vi "Dryer PreCondition SM.vi"(0 "Equipment":T1, 1 "CDAQ Tasks":refnum<k21>[](array[refnum]), 5 "RDB Channel":string="1001", 7 "Power On Threshold":dbl=50.0, 9 "CDAQ?":bool, 11 "Error In":errorcluster) -> (4 "Cold Dryer Weight":dbl, 15 "Error Out":errorcluster)   [LabVIEW 2012]
uses:
  Equipment DPT.ctl
  WT500/WT500 Sequences.ctl
  Global Test Variables DPT.vi
  <vilib>/Analysis/baseanly.llb/Mean (DBL).vi
  Drivers/Agilent 34970/Agilent 34970.lvlib
  <vilib>/Analysis/NI_AALBase.lvlib
panel:
  out "Debug State":string[](array[string])
  in  "Tab Control":enum32{"Page 1", "Page 2"}(tab)
  out "CDAQ Data Out":dbl[](array[numeric])
  out "15 min Up":bool
  out "Temp stable":bool
  out "Current State":string
  in  "Debug?":bool=TRUE
  in  "10 Min":i32=600
  in  "5min":dbl=300.0
  out "Test Setup.RH-IP":string
  out "Test AG Chan List":string
  out "Saved Channel List":string
  out "Agilent Error Message":string
  out "Timer":dbl format="%<%H:%M:%S>t"
  out "Temperature-RDB":dbl(graph)
  out "RDB (F)":dbl
  out "Ambient Temp(F)":dbl
  out "RH":dbl
  out "Power":dbl
  out "String":string
  in  "Exit":bool
  # "Before any test cycle, operate the dryer without a test load in the non-heat mode for 15 minutes\nor until the discharge air temperature is varying less than 1 °F for 10 minutes, which ever is longer, in the test installation location\nwith the ambient conditions within the specified rest condition tolerances of 2.2."
  # "2.2 Ambient temperature and humidity. Maintain the room ambient air temperature at 75 ±3 °F and the room relative humidity at 50\n±10 percent relative humidity"
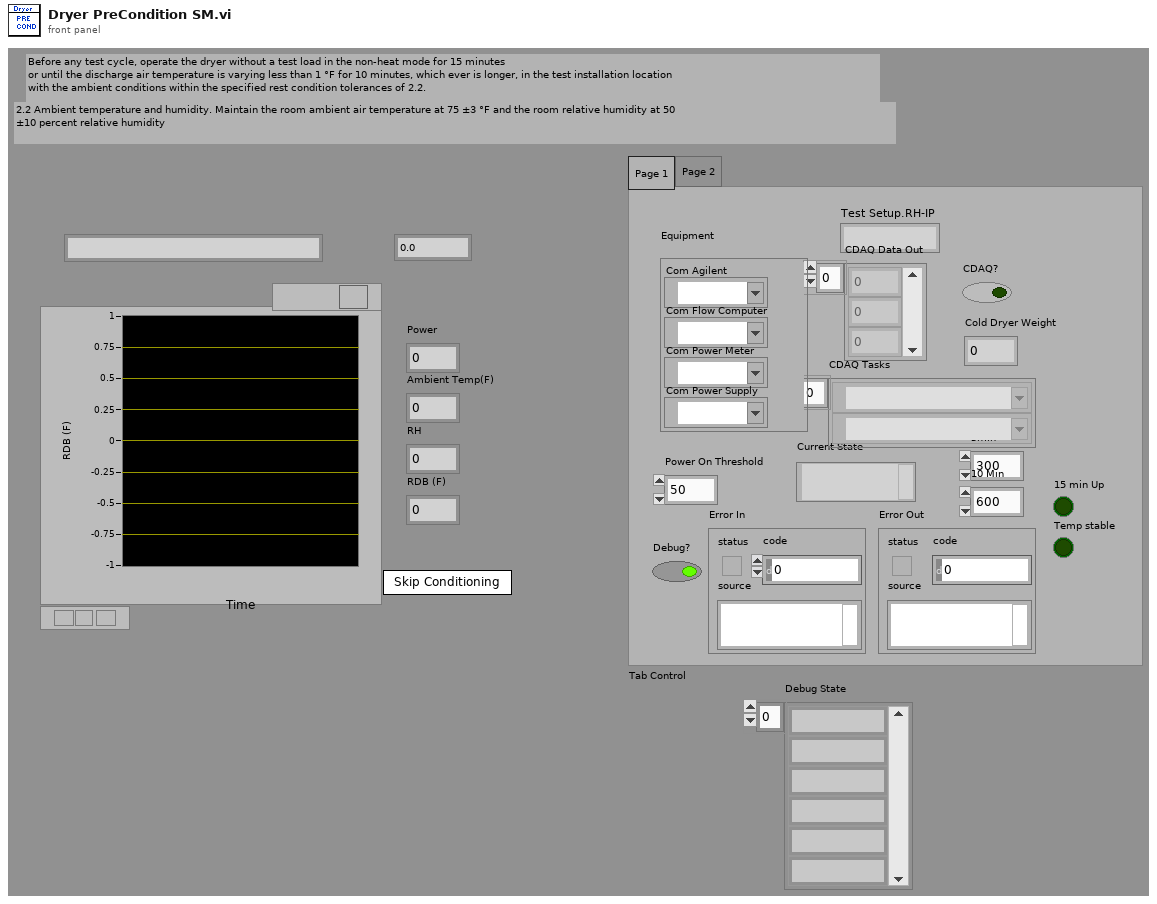
[diagram p1: front panel]
types:
  T1 = typedef "Equipment DPT.ctl" = cluster{"Com Agilent":refnum<visa-resource-name>, "Com Flow Computer":refnum<visa-resource-name>, "Com Power Meter":refnum<visa-resource-name>, "Com Power Supply":refnum<visa-resource-name>}
  T2 = enum32{"invalid app kind", "Development System", "Run Time System", "Student Edition", "Embedded LabVIEW", "Evaluation", "Custom"}
  T3 = enum16{"Exe", "Init CDAQ", "Gather DATA", "Close"}
  T4 = enum32{"Invalid", "Standard", "Closed", "Hidden", "Minimized", "Maximized"}
  T5 = typedef "WT500 Sequences.ctl" = enum16{"Initialize", "GetReadings", "GetErrors", "Close", "NoOp", "MiscCmd"}
  T6 = cluster{"Core":cluster{"Current VI Reference":refnum<vi>, "Close Panel on Exit?":bool}, "Agilent Channel List":string, "Equipment":T1, "Power On Threshold":dbl, "RDB Channel":string, "T0":dbl, "Tstart":dbl, "Temps":dbl[], "CDAQ?":bool, "CDAQ Tasks":refnum<k21>[]}
  T7 = cluster{"Current VI Reference":refnum<vi>, "Close Panel on Exit?":bool}
  T8 = typedef "DPT Global Type.ctl" = cluster{"Test Setup":cluster{"RH Resistor":dbl, "Temp Cal":dbl, "Temp Coeff":dbl, "Power On Threshold":dbl, "MA Filter Size":i32, "Weight Offset":dbl, "Temp Resistor":dbl, "Gas Enabled":bool, "Gas P. Resistor":dbl, "Scale Com":dbl, "W. Samps":i32, "Temp4mA Val":dbl, "Temp20mA Val":dbl, "RH4mA Val":dbl, "RH20mA Val":dbl, "GPres4mA Val":dbl, "Gpres20mA Val":dbl, "Smoothing":bool, "CDAQ":bool, "34970":bool, "34980":bool, "RH-IP":string, "RH-IP2":string, "RH-IP3":string, "CompVolume":dbl, "T45_Coeff.":dbl}, "Agilent Setup":cluster{"Scale Channel":string, "TC Channels":string, "VDC Discrete Channels":string, "RH Chan":string, "Temp Chan":string, "Tscale Channel":string, "RDB Channel":string, "Gas Temperature":string, "Gas Pressure":string, "Barometric Pressure":string, "Gas Feedback Chan":string}, "Directories":cluster{"Work File Directory":path, "Save File Directory":path, "Library Directory":path, "Data Backup Directory":path, "Data Backup Dir Fail":path, "Lab Directory":path}, "Test Information":cluster{"Model:":string, "Temperature:":string, "Engineer:":string, "Technician:":string, "Comments:":string, "Lab ID:":string, "TR Number:":string, "Test Number:":string, "Test Station:":string, "Empty Dryer Cold Weight:":dbl, "Serial Number:":string, "Build:":string, "Dryer Type":string, "Humidity":string, "Test Title per TR:":string}, "cDAQ Array Locations":cluster{"Scale Channel":string, "TC Channels":string, "VDC Discrete Channel":string, "RH Chan":string, "Temp Chan":string, "Tscale Channel":string, "RDB Channel":string, "Gas Temperature":string, "Gas Pressure":string, "Barometric Pressure":string, "Gas Feedback Chan":string}}
  T9 = typedef "Dryer PowerData.ctl" = cluster{"Current L1":dbl, "Current L2":dbl, "Power":dbl, "WattHours":dbl}
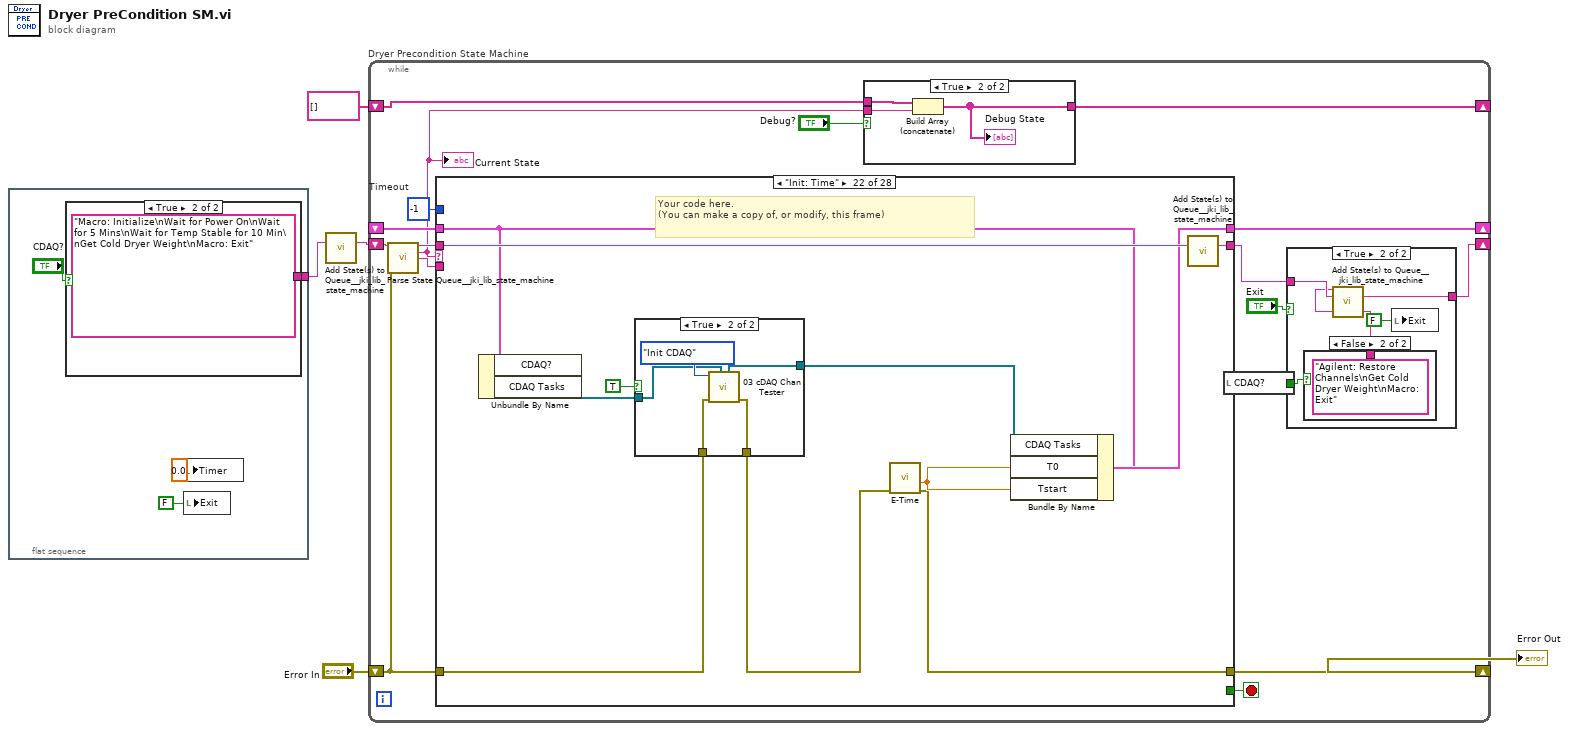
[diagram p0: block diagram]
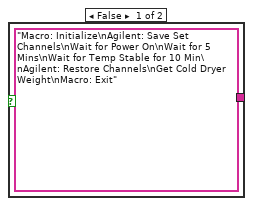
[diagram p2: hidden frame]
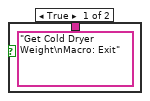
[diagram p5: hidden frame]
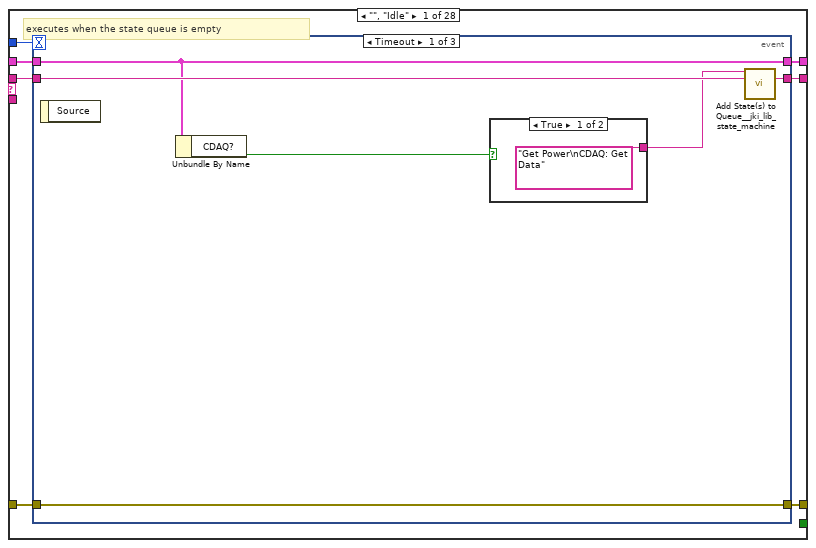
[diagram p6: hidden frame]
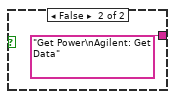
[diagram p7: hidden frame]
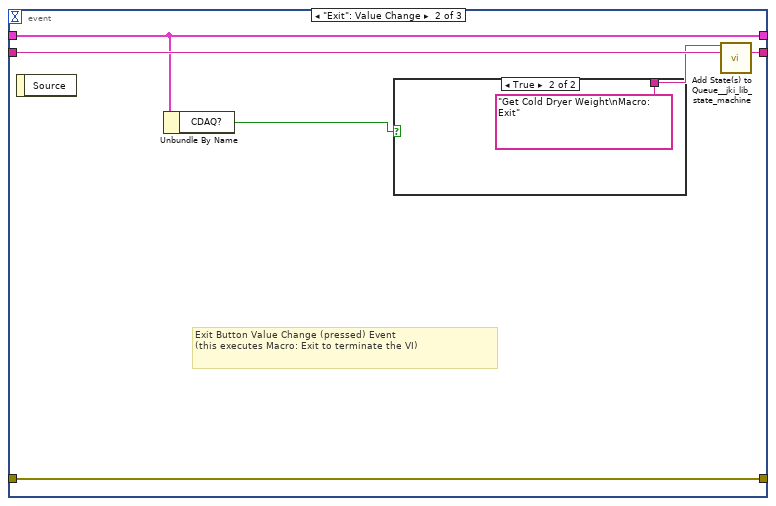
[diagram p8: hidden frame]
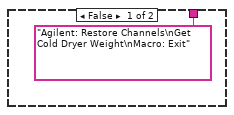
[diagram p9: hidden frame]
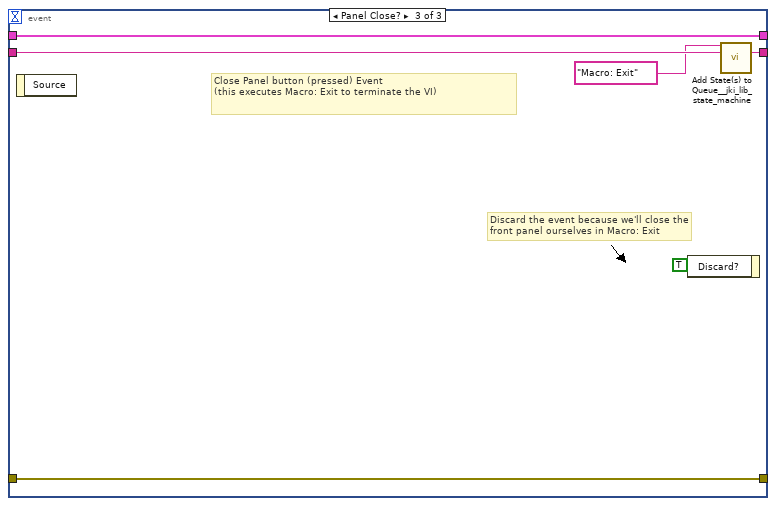
[diagram p10: hidden frame]
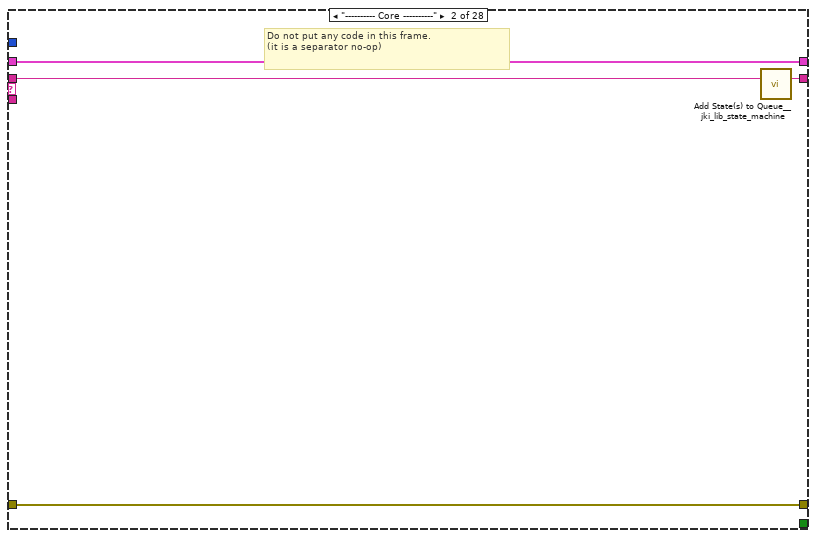
[diagram p11: hidden frame]
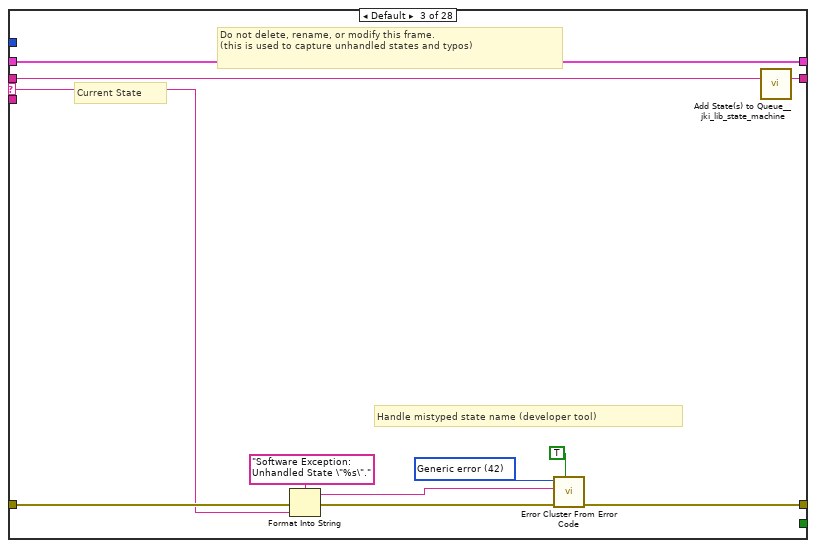
[diagram p12: hidden frame]
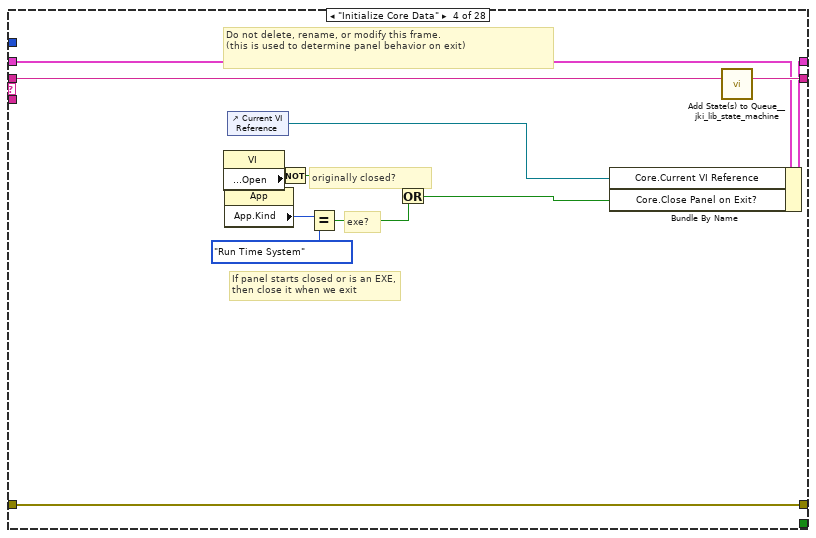
[diagram p13: hidden frame]
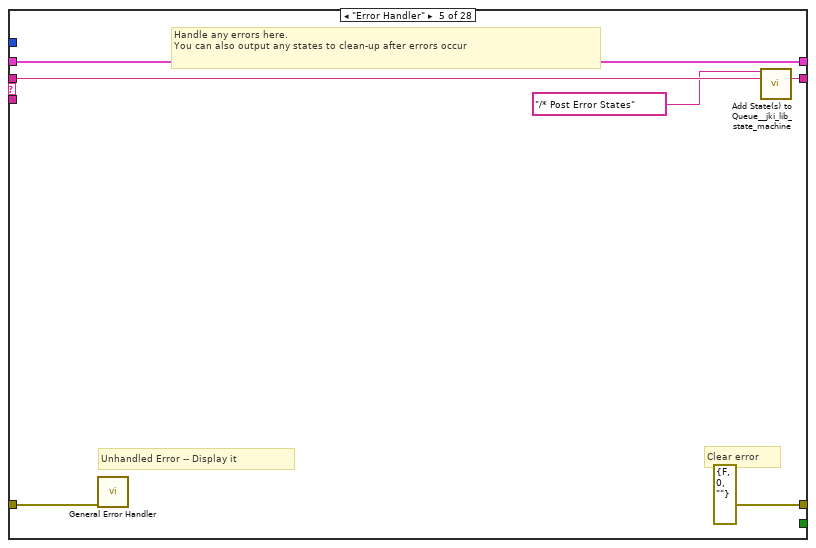
[diagram p14: hidden frame]
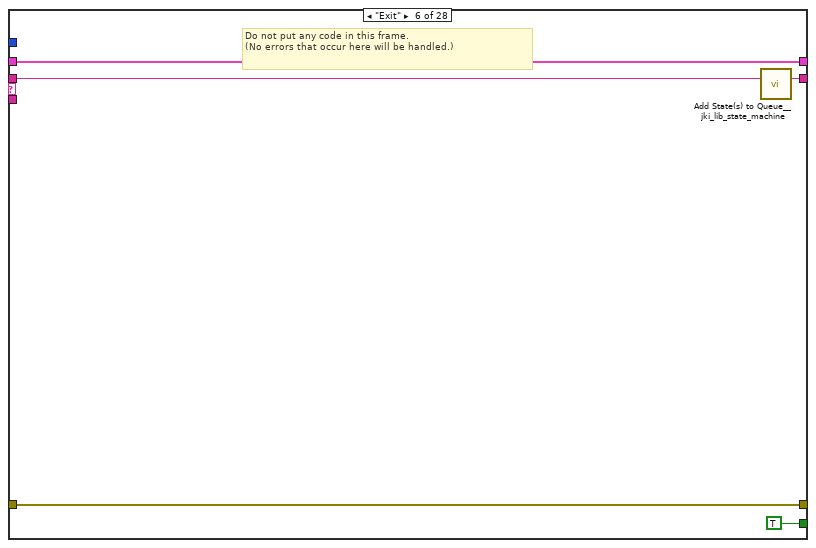
[diagram p15: hidden frame]
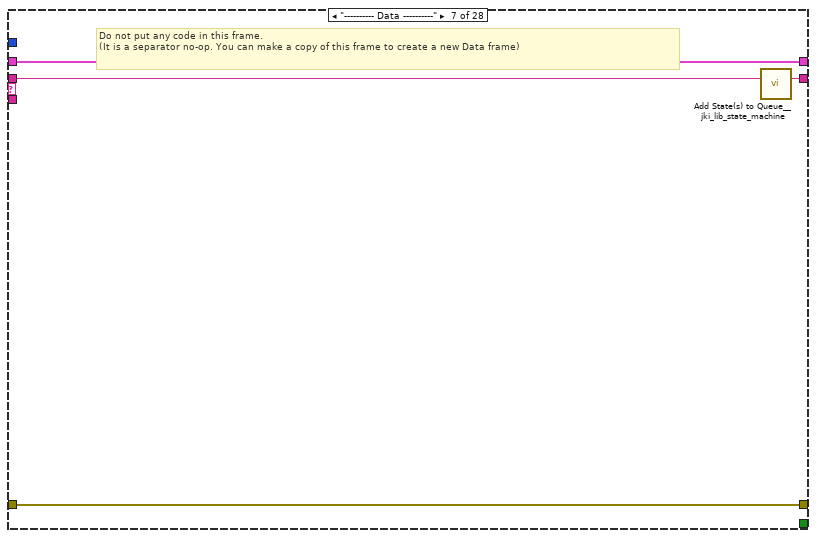
[diagram p16: hidden frame]
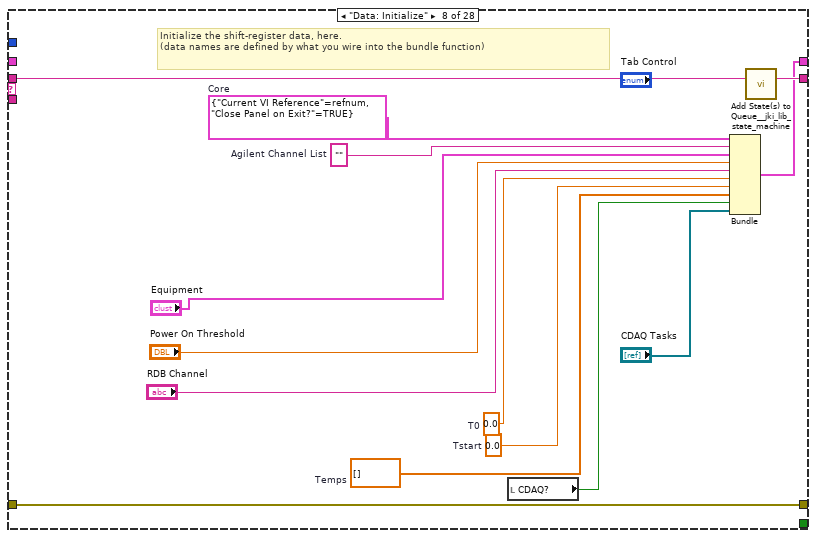
[diagram p17: hidden frame]
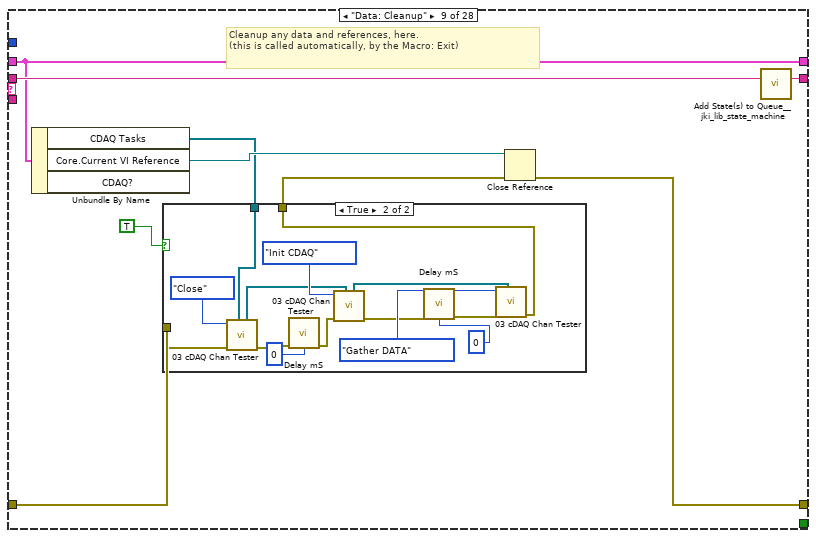
[diagram p18: hidden frame]
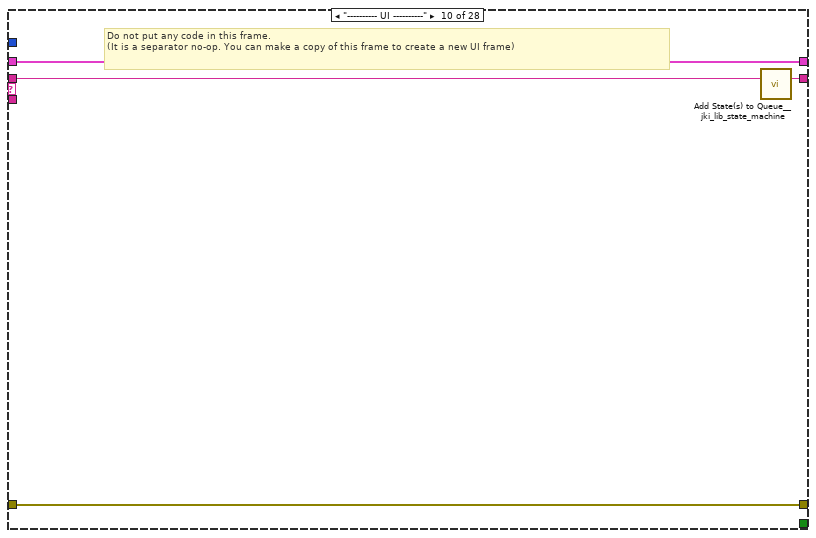
[diagram p20: hidden frame]
diagram:
  n1 = flat-sequence {
    tunnel: [w9] -> w4
    frame #0 {
      n2 = case shown="True" "CDAQ?" {
        tunnel: ["Macro: Initialize\nAgilent: Save Set Channels\nWait for Power On\nWait for 5 Mins\nWait for Temp Stable for 10 Min\nAgilent: Restore Channels\nGet Cold Dryer Weight\nMacro: Exit" "Macro: Initialize\nWait for Power On\nWait for 5 Mins\nWait for Temp Stable for 10 Min\nGet Cold Dryer Weight\nMacro: Exit"] -> w9
        frame False {
        }
        frame True {
        }
      }
      n3 = local write "Timer"(0.0 ("Timer")) -> ()
      n4 = local write "Exit"(FALSE ("Exit")) -> ()
    }
  }
  n5 = call <vilib>:"Add State(s) to Queue__jki_lib_state_machine.vi"("State(s) in (\"\")"=w4) -> ("States Out"=w5:string)  [unwired: 14 in]
  n6 = while "Dryer Precondition State Machine" {
    shift-right: [w23] -> _
    shift-left: _ -> [w22]
    shift-right: [w25] -> w2
    shift-left: "Error In" -> [w20]
    shift-right: [w18] -> _
    shift-left: w5 -> [w26]
    shift-right: [w13] -> _
    shift-left: string[] [] -> [w12]
    stop <- w24 stop-if-true
    w21 = -1  # Timeout
    n7 = call <vilib>:"Parse State Queue__jki_lib_state_machine.vi"("State Queue"=w26, "Error In (no error)"=w20) -> ("Remaining States"=w28:string, "Current State"=w14:string, "Arguments"=w27:string)  [unwired: 11 in]
    "Current State" <- w14
    n8 = case shown="\"Init: Time\"" w14 {
      selector: w14 -> [_ _ w74 _ _ _ _ _ _ _ _ _ _ _ _ _ _ _ _ _ _ _ _ _ _ _ _ _]
      tunnel: w28 -> [w47 w73 w78 w96 w102 w107 w111 w125 w134 w153 w157 w163 w174 w200 w205 w215 w219 w231 w260 w290 w343 w371 w387 w410 w481 w497 w509 w516]
      tunnel: w27 -> [_ _ _ _ _ _ _ _ _ _ _ w158 w168 _ _ _ _ _ _ _ _ _ _ _ _ _ _ _]
      tunnel: w22 -> [w45 w70 w76 w87 w99 w105 w108 _ w130 w150 w155 w161 w170 w197 w202 w212 w216 w227 w257 w287 w334 w366 w383 w406 w466 w495 w502 w514]
      tunnel: [w44 w71 w80 w93 errorcluster {"status"=FALSE, "code"=0, "source"=""} ("error out") w104 w109 w123 w131 w151 w154 w159 w171 w198 w203 w213 w217 w228 w258 w288 w330 w367 w384 w397 w464 w493 w503 w510] -> w25
      tunnel: w20 -> [w43 w71 w79 w93 w98 w104 w109 w123 w129 w151 w154 w160 w172 w198 w203 w213 w217 w228 w258 w288 w333 w365 w385 w405 w479 w494 w504 w510]
      tunnel: [w46 w72 w77 w95 w101 w106 w110 w124 w133 w152 w156 w162 w173 w199 w204 w214 w218 w230 w259 w289 w342 w370 w386 w409 w480 w496 w508 w515] -> w19
      tunnel: [_ _ _ _ _ TRUE _ _ _ _ _ _ _ _ _ _ _ _ _ _ _ _ _ _ _ _ _ _] -> w24
      tunnel: [w42 w70 w76 w94 w99 w105 w108 w118 w130 w150 w155 w161 w170 w197 w202 w212 w216 w226 w256 w286 w336 w369 w383 w406 w466 w495 w502 w514] -> w23
      tunnel: w21 -> [w41 _ _ _ _ _ _ _ _ _ _ _ _ _ _ _ _ _ _ _ _ _ _ _ _ _ _ _]
      frame "", "Idle" {
        # "executes when the state queue is empty"
        n9 = event shown="[0] Timeout" {
          selector: _ -> [_ _ _]
          dyn-events: _ -> [_ _ _]
          timeout: w41 -> [_ _ _]
          tunnel: w47 -> [w53 w61 w69]
          tunnel: [w52 w60 w68] -> w46
          tunnel: w45 -> [w49 w57 w66]
          tunnel: [w51 w59 w67] -> w44
          tunnel: w43 -> [w51 w59 w67]
          tunnel: [w49 w57 w66] -> w42
          event Timeout {
            n10 = event-data() -> ()  [unwired: 1 in, 1 out]
            n11 = Unbundle By Name(w49) -> ("CDAQ?"=w48:bool)
            n12 = case shown="True" w48 {
              tunnel: ["Get Power\nCDAQ: Get Data" ("State(s) in Front (\"\")") "Get Power\nAgilent: Get Data" ("State(s) in Front (\"\")")] -> w50
              frame True {
              }
              frame False {
              }
            }
            n13 = call <vilib>:"Add State(s) to Queue__jki_lib_state_machine.vi"("State(s) in Front (\"\")"=w50, "State(s) in (\"\")"=w53) -> ("States Out"=w52:string)  [unwired: 13 in]
          }
          event "Exit": Value Change {
            # "Exit Button Value Change (pressed) Event\n(this executes Macro: Exit to terminate the VI)"
            n14 = event-data() -> ()  [unwired: 1 in, 1 out]
            n15 = Unbundle By Name(w57) -> ("CDAQ?"=w56:bool)
            n16 = case shown="True" w56 {
              tunnel: ["Agilent: Restore Channels\nGet Cold Dryer Weight\nMacro: Exit" "Get Cold Dryer Weight\nMacro: Exit"] -> w58
              frame False {
              }
              frame True {
              }
            }
            n17 = call <vilib>:"Add State(s) to Queue__jki_lib_state_machine.vi"("State(s) in Front (\"\")"=w58, "State(s) in (\"\")"=w61) -> ("States Out"=w60:string)  [unwired: 13 in]
          }
          event Panel Close? {
            # "Discard the event because we'll close the front panel ourselves in Macro: Exit"
            # "Close Panel button (pressed) Event\n(this executes Macro: Exit to terminate the VI)"
            n18 = event-data() -> ()  [unwired: 1 in, 1 out]
            n19 = event-data("Discard?"=TRUE) -> ()  [unwired: 1 in, 1 out]
            n20 = call <vilib>:"Add State(s) to Queue__jki_lib_state_machine.vi"("State(s) in Front (\"\")"="Macro: Exit", "State(s) in (\"\")"=w69) -> ("States Out"=w68:string)  [unwired: 13 in]
          }
        }
      }
      frame "---------- Core ----------" {
        # "Do not put any code in this frame.\n(it is a separator no-op)"
        n21 = call <vilib>:"Add State(s) to Queue__jki_lib_state_machine.vi"("State(s) in (\"\")"=w73) -> ("States Out"=w72:string)  [unwired: 14 in]
      }
      frame Default {
        w83 = 42 items=["No error", "Argument error", "Memory is full", "Out of zone", "End of file", "File already open", "Generic file I/O error", "File not found", "File permission error", "Disk is full", "Duplicate path", "Too many files open", "System feature not enabled", "Resource file not found", "Cannot add resource", "Resource not found", "Image not found", "Image memory error", "Pen does not exist", "Config type invalid", "Config token not found", "Config parse error", "Config memory error", "Bad external code format", "Bad external code offset", "External code not present", "Null window", "Destroy window error", "Null menu", "Print aborted", "Bad print record", "Print driver error", "Windows error during printing", "Memory error during printing", "Print dialog error", "Generic print error", "Invalid device refnum", "Device not found", "Device parameter error", "Device unit error", "Cannot open device", "Device call aborted", "Generic error", "Cancelled by user", "Object ID too low", "Object ID too high", "Object not in heap", "Unknown heap", "Unknown object (invalid DefProc)", "Unknown object (DefProc not in table)", "Message out of range", "Invalid (null) method", "Unknown message", "Manager call not supported", "Bad address", "Network operation in progress", "Network operation timed out", "Connection is busy", "Network attribute not supported", "Network error", "Address in use", "System out of memory", "Connection aborted", "Connection refused", "Not connected", "Already connected", "Connection closed", "Initialization error (interapplication manager)", "Bad occurrence", "Wait on unbound occurrence handler", "Occurrence queue overflow", "Datalog type conflict", "Unused", "Unrecognized type (interapplication manager)", "Memory corrupt", "Failed to make temporary DLL", "Old CIN version", "Drag socket not found", "Failed to load drop-object", "Failed to register OLE object", "Failed to release OLE object", "Format specifier type mismatch", "Unknown format specifier", "Too few format specifiers", "Too many format specifiers", "Scan failed", "Newer CIN version", "Error converting to variant", "Runtime menu error", "Password tampered", "Variant attribute not found", "Incompatible variant data type", "Event data is not available", "Event Store is not present", "Occurrence is not found", "Event Queue is not created", "Event info is not available", "Refnum passed is NULL", "Error retrieving Class GUID", "Error retrieving CoClass GUID", "Error retrieving TypeLib GUID.", "Bad built application magic bytes.", "Specific driver is different from the specific driver associated with the Logical Name.", "There is no session opened to the class driver.", "Max Error", "MAX - Error with config objects", "MAX - Error loading configuration", "MAX - Group not supported"]
        # "Current State"
        # "Do not delete, rename, or modify this frame.\n(this is used to capture unhandled states and typos)"
        # "Handle mistyped state name (developer tool)"
        n22 = Format Into String(format string="Software Exception: Unhandled State \"%s\"." ("message"), error in=w79, w74) -> (resulting string=w82:string, error out=w81:errorcluster)  [unwired: 1 in]
        n23 = call <vilib>:"Error Cluster From Error Code.vi"("show call chain? (False)"=TRUE, "error in (no error)"=w81, "error message (\"\")"=w82, "error code (0)"=w83) -> ("error out"=w80:errorcluster)  [unwired: 5 in]
        n24 = call <vilib>:"Add State(s) to Queue__jki_lib_state_machine.vi"("State(s) in (\"\")"=w78) -> ("States Out"=w77:string)  [unwired: 14 in]
      }
      frame "Initialize Core Data" {
        # "Do not delete, rename, or modify this frame.\n(this is used to determine panel behavior on exit)"
        # "originally closed?"
        # "exe?"
        # "If panel starts closed or is an EXE, then close it when we exit"
        n25 = property class="VI"() -> ("Front Panel.Open"=w92:bool)  [unwired: 2 in, 2 out]
        n26 = property class="App"() -> ("App.Kind"=w91:T2)  [unwired: 2 in, 2 out]
        n27 = control-ref of="Current VI Reference"() -> (w85:refnum<vi>)
        n28 = Not(x=w92) -> (.not. x?=w89:bool)
        n29 = Equal?(x=w91, y=T2."Run Time System" ("Application:Kind")) -> (x = y?=w88:bool)
        n30 = Or(x=w89, y=w88) -> (x .or. y?=w86:bool)
        n31 = Bundle By Name(cluster=w87, "Core.Current VI Reference"=w85, "Core.Close Panel on Exit?"=w86) -> (w94:T6)
        n32 = call <vilib>:"Add State(s) to Queue__jki_lib_state_machine.vi"("State(s) in (\"\")"=w96) -> ("States Out"=w95:string)  [unwired: 14 in]
      }
      frame "Error Handler" {
        # "Unhandled Error -- Display it"
        # "Handle any errors here.\nYou can also output any states to clean-up after errors occur"
        # "Clear error"
        n33 = call <vilib>:"General Error Handler.vi"("error in (no error)"=w98) -> ()  [unwired: 10 in, 5 out]
        n34 = call <vilib>:"Add State(s) to Queue__jki_lib_state_machine.vi"("State(s) in Front (\"\")"="/* Post Error States", "State(s) in (\"\")"=w102) -> ("States Out"=w101:string)  [unwired: 13 in]
      }
      frame "Exit" {
        # "Do not put any code in this frame.\n(No errors that occur here will be handled.)"
        n35 = call <vilib>:"Add State(s) to Queue__jki_lib_state_machine.vi"("State(s) in (\"\")"=w107) -> ("States Out"=w106:string)  [unwired: 14 in]
      }
      frame "---------- Data ----------" {
        # "Do not put any code in this frame.\n(It is a separator no-op. You can make a copy of this frame to create a new Data frame)"
        n36 = call <vilib>:"Add State(s) to Queue__jki_lib_state_machine.vi"("State(s) in (\"\")"=w111) -> ("States Out"=w110:string)  [unwired: 14 in]
      }
      frame "Data: Initialize" {
        w114 = dbl[] []  # Temps
        w115 = 0.0  # Tstart
        w116 = 0.0  # T0
        w119 = ""  # Agilent Channel List
        w122 = T7 {"Current VI Reference"=refnum, "Close Panel on Exit?"=TRUE}  # Core
        # "Initialize the shift-register data, here.\n(data names are defined by what you wire into the bundle function)"
        n37 = local read "CDAQ?"() -> (w113:bool)
        n38 = Bundle("Core"=w122, "Agilent Channel List"=w119, "Equipment"="Equipment", "Power On Threshold"="Power On Threshold", "RDB Channel"="RDB Channel", "T0"=w116, "Tstart"=w115, "Temps"=w114, "CDAQ?"=w113, "CDAQ Tasks"="CDAQ Tasks") -> (w118:T6)  [unwired: 1 in]
        n39 = call <vilib>:"Add State(s) to Queue__jki_lib_state_machine.vi"("State(s) in (\"\")"=w125) -> ("States Out"=w124:string)  [unwired: 14 in]
      }
      frame "Data: Cleanup" {
        # "Cleanup any data and references, here.\n(this is called automatically, by the Macro: Exit)"
        n40 = Unbundle By Name(w130) -> ("CDAQ Tasks"=w127:refnum<k21>[], "Core.Current VI Reference"=w132:refnum<vi>)  [unwired: 1 out]
        n41 = case shown="True" TRUE {
          tunnel: w129 -> [w135 w149]
          tunnel: [w135 w140] -> w128
          tunnel: w127 -> [_ w147]
          frame False {
          }
          frame True {
            n42 = call "03 cDAQ Chan Tester.vi"("Tasks In"=w147, "error in (no error)"=w149, "Mode"=T3."Close") -> ("error out"=w145:errorcluster, "Tasks Out"=w142:refnum<k21>[])  [unwired: 6 in, 1 out]
            n43 = call "Delay mS.vi"("Error In"=w145, "milliseconds to wait"=u32 0) -> ("Error Out"=w146:errorcluster)  [unwired: 13 in]
            n44 = call "03 cDAQ Chan Tester.vi"("Tasks In"=w142, "error in (no error)"=w146, "Mode"=T3."Init CDAQ") -> ("error out"=w138:errorcluster, "Tasks Out"=w141:refnum<k21>[])  [unwired: 6 in, 1 out]
            n45 = call "Delay mS.vi"("Error In"=w138, "milliseconds to wait"=u32 0) -> ("Error Out"=w137:errorcluster)  [unwired: 13 in]
            n46 = call "03 cDAQ Chan Tester.vi"("Tasks In"=w141, "error in (no error)"=w137, "Mode"=T3."Gather DATA") -> ("error out"=w140:errorcluster)  [unwired: 6 in, 2 out]
          }
        }
        n47 = Close Reference(reference=w132, error in (no error)=w128) -> (error out=w131:errorcluster)
        n48 = call <vilib>:"Add State(s) to Queue__jki_lib_state_machine.vi"("State(s) in (\"\")"=w134) -> ("States Out"=w133:string)  [unwired: 14 in]
      }
      frame "---------- UI ----------" {
        # "Do not put any code in this frame.\n(It is a separator no-op. You can make a copy of this frame to create a new UI frame)"
        n49 = call <vilib>:"Add State(s) to Queue__jki_lib_state_machine.vi"("State(s) in (\"\")"=w153) -> ("States Out"=w152:string)  [unwired: 14 in]
      }
      frame "UI: Initialize" {
        # "Initialize the User Interface, here.\n(this is called automatically, by the Macro: Init)"
        n50 = call <vilib>:"Add State(s) to Queue__jki_lib_state_machine.vi"("State(s) in (\"\")"=w157) -> ("States Out"=w156:string)  [unwired: 14 in]
      }
      frame "UI: Cursor Set" {
        # "Argument"
        # "Set and Unset Cursor Busy.\n(Usage: \"UI: Cursor Set >> Busy|Idle\")"
        n51 = case shown="\"Idle\", Default" w158 {
          tunnel: w160 -> [w165 w167]
          tunnel: [w164 w166] -> w159
          frame "Idle", Default {
            n52 = call <vilib>:"Unset Busy.vi"("error in (no error)"=w165) -> ("error out"=w164:errorcluster)  [unwired: 10 in]
          }
          frame "Busy" {
            n53 = call <vilib>:"Set Busy.vi"("error in (no error)"=w167) -> ("error out"=w166:errorcluster)  [unwired: 9 in, 1 out]
          }
        }
        n54 = call <vilib>:"Add State(s) to Queue__jki_lib_state_machine.vi"("State(s) in (\"\")"=w163) -> ("States Out"=w162:string)  [unwired: 14 in]
      }
      frame "UI: Front Panel State" {
        # "Argument"
        # "Set Front Panel Open or Closed\n(Usage: \"UI: Front Panel State >> Open|Close\")"
        n55 = Unbundle By Name(w170) -> ("Core.Current VI Reference"=w169:refnum<vi>)
        n56 = case shown="\"Open\", Default" w168 {
          tunnel: w172 -> [w178 w191]
          tunnel: [w180 w192] -> w171
          tunnel: w169 -> [w179 w189]
          frame "Open", Default {
            n57 = property class="VI"(reference=w179, error in=w178) -> (reference out=w176:refnum<vi>, error out=w177:errorcluster, "Front Panel.Open"=w175:bool)
            n58 = case shown="False" w175 {
              tunnel: [w183 w186] -> w180
              tunnel: w177 -> [w182 w186]
              tunnel: w176 -> [w181 _]
              frame False {
                n59 = invoke class="VI" method="FP.Open"(reference=w181, error in=w182, "Activate"=TRUE, "State"=T4."Standard") -> (error out=w183:errorcluster)  [unwired: 1 in, 4 out]
              }
              frame True {
              }
            }
          }
          frame "Close" {
            n60 = property class="VI"(reference=w189, error in=w191) -> (reference out=w188:refnum<vi>, error out=w190:errorcluster, "Front Panel.Open"=w187:bool)
            n61 = case shown="True" w187 {
              tunnel: [w193 w196] -> w192
              tunnel: w190 -> [w193 w195]
              tunnel: w188 -> [_ w194]
              frame False {
              }
              frame True {
                n62 = invoke class="VI" method="FP.Close"(reference=w194, error in=w195) -> (error out=w196:errorcluster)  [unwired: 1 in, 2 out]
              }
            }
          }
        }
        n63 = call <vilib>:"Add State(s) to Queue__jki_lib_state_machine.vi"("State(s) in (\"\")"=w174) -> ("States Out"=w173:string)  [unwired: 14 in]
      }
      frame "---------- Macro ----------" {
        # "Do not put any code in this frame.\n(It is a separator no-op. You can make a copy of this frame to create a new Macro frame)"
        n64 = call <vilib>:"Add State(s) to Queue__jki_lib_state_machine.vi"("State(s) in (\"\")"=w200) -> ("States Out"=w199:string)  [unwired: 14 in]
      }
      frame "Macro: Initialize" {
        w201 = "Data: Initialize\nInit: Time\nInitialize Core Data\nUI: Initialize\nUI: Front Panel State >> Open"  # Data: Initialize Init: Time Initialize Core Data UI: Initialize UI: Front Panel State >> Open
        # "Initialization Macro\n(This is called once, when the VI starts)"
        n65 = call <vilib>:"Add State(s) to Queue__jki_lib_state_machine.vi"("State(s) in Front (\"\")"=w201, "State(s) in (\"\")"=w205) -> ("States Out"=w204:string)  [unwired: 13 in]
      }
      frame "Macro: Exit" {
        # "Exit Macro\n(This is called once, when the VI exits)"
        n66 = Unbundle By Name(w212) -> ("Core.Close Panel on Exit?"=w211:bool)
        n67 = Select(t="UI: Front Panel State >> Close", s=w211, f="") -> (s? t:f=w208:string)
        n68 = call <vilib>:"Add State(s) to Queue__jki_lib_state_machine.vi"("State(s) in (\"\")"=w208, "State(s) at Back (\"\")"="Data: Cleanup\nExit") -> ("States Out"=w206:string)  [unwired: 13 in]
        n69 = call <vilib>:"Add State(s) to Queue__jki_lib_state_machine.vi"("State(s) in Front (\"\")"=w206, "State(s) in (\"\")"=w215) -> ("States Out"=w214:string)  [unwired: 13 in]
      }
      frame "----------Test ----------" {
        # "Template Separator\n(You can make a copy of, or modify, this frame)"
        n70 = call <vilib>:"Add State(s) to Queue__jki_lib_state_machine.vi"("State(s) in (\"\")"=w219) -> ("States Out"=w218:string)  [unwired: 14 in]
      }
      frame "Wait for Power On" {
        # "Your code here.\n(You can make a copy of, or modify, this frame)"
        n71 = Unbundle By Name(w227) -> ("CDAQ?"=w220:bool, "Tstart"=w224:dbl, "Power On Threshold"=w223:dbl)
        n72 = local read "Power"() -> (w222:dbl)
        n73 = Greater?(x=w223, y=w222) -> (0:w221:bool)
        n74 = case shown="True" w221 {
          tunnel: w227 -> [w233 w242]
          tunnel: [w233 w241] -> w226
          tunnel: ["" ("State(s) in Front (\"\")") w239] -> w225
          tunnel: w224 -> [_ w236]
          tunnel: w220 -> [_ w234]
          frame False {
          }
          frame True {
            n75 = call "E-Time.vi"() -> ("Elapsed Time (sec)"=w243:dbl)  [unwired: 9 in, 2 out]
            n76 = call "Timeout Calc.vi"("Complete time"=w243, "Gather Data Period"=1000, "Start Time"=w236) -> ("Delay Time"=w238:i32)  [unwired: 8 in]
            n77 = event shown="[0] Timeout" {
              selector: _ -> [_]
              dyn-events: _ -> [_]
              timeout: w238 -> [_]
              tunnel: [w245] -> w240
              tunnel: [w246] -> w239
              tunnel: [w245] -> w235
              tunnel: w234 -> [w244]
              event Timeout {
                n78 = event-data() -> ()  [unwired: 1 in, 2 out]
                n79 = case shown="True" w244 {
                  tunnel: ["Get Power\nCDAQ: Get Data\nWait for Power On" ("State(s) in Front (\"\")") "Get Power\nAgilent: Get Data\nWait for Power On" ("State(s) in Front (\"\")")] -> w246
                  frame True {
                  }
                  frame False {
                  }
                }
                n80 = call "E-Time.vi"() -> ("Elapsed Time (sec)"=w245:dbl)  [unwired: 9 in, 2 out]
              }
            }
            n81 = Bundle By Name(cluster=w242, "Tstart"=w240, "T0"=w235) -> (w241:T6)
          }
        }
        n82 = call <vilib>:"Add State(s) to Queue__jki_lib_state_machine.vi"("State(s) in Front (\"\")"=w225, "State(s) in (\"\")"=w231) -> ("States Out"=w230:string)  [unwired: 13 in]
        "String" <- "Start Fluffing: Waiting for Power ON"
      }
      frame "Wait for 5 Mins" {
        # "Your code here.\n(You can make a copy of, or modify, this frame)"
        n83 = Unbundle By Name(w257) -> ("Tstart"=w254:dbl, "CDAQ?"=w249:bool)
        n84 = local read "Timer"() -> (w252:dbl)
        n85 = Greater?(x=w252, y="5min") -> (0:w253:bool)
        n86 = case shown="False" w253 {
          tunnel: w257 -> [w268 w276]
          tunnel: [w267 w276] -> w256
          tunnel: [w265 "" ("State(s) in Front (\"\")")] -> w255
          tunnel: w254 -> [w262 _]
          tunnel: w249 -> [w261 _]
          frame False {
            n87 = call "E-Time.vi"() -> ("Elapsed Time (sec)"=w269:dbl)  [unwired: 9 in, 2 out]
            n88 = call "Timeout Calc.vi"("Complete time"=w269, "Gather Data Period"=1000, "Start Time"=w262) -> ("Delay Time"=w264:i32)  [unwired: 8 in]
            n89 = event shown="[0] Timeout" {
              selector: _ -> [_]
              dyn-events: _ -> [_]
              timeout: w264 -> [_]
              tunnel: [w272] -> w266
              tunnel: [w271] -> w265
              tunnel: w261 -> [w270]
              event Timeout {
                n90 = event-data() -> ()  [unwired: 1 in, 2 out]
                n91 = case shown="True" w270 {
                  tunnel: ["Post Time\nGet Power\nCDAQ: Get Data\nWait for 5 Mins" ("State(s) in Front (\"\")") "Post Time\nGet Power\nAgilent: Get Data\nWait for 5 Mins" ("State(s) in Front (\"\")")] -> w271
                  frame True {
                  }
                  frame False {
                  }
                }
                n92 = call "E-Time.vi"() -> ("Elapsed Time (sec)"=w272:dbl)  [unwired: 9 in, 2 out]
              }
            }
            n93 = Bundle By Name(cluster=w268, "Tstart"=w266) -> (w267:T6)
          }
          frame True {
          }
        }
        n94 = local write "String"("Air Fluffing...") -> ()
        n95 = call <vilib>:"Add State(s) to Queue__jki_lib_state_machine.vi"("State(s) in Front (\"\")"=w255, "State(s) in (\"\")"=w260) -> ("States Out"=w259:string)  [unwired: 13 in]
      }
      frame "Wait for Temp Stable for 10 Min" {
        # "Your code here.\n(You can make a copy of, or modify, this frame)"
        n96 = Unbundle By Name(w287) -> ("CDAQ?"=w277:bool, "Tstart"=w284:dbl, "Temps"=w278:dbl[])
        n97 = Array Size(array=w278) -> (size(s)=w282:i32)
        n98 = Greater?(x=w282, y="10 Min") -> (0:w280:bool)
        "15 min Up" <- w280
        n99 = case shown="True" w280 {
          selector: w280 -> [w291 _]
          tunnel: [w291 w292] -> w279
          tunnel: w278 -> [_ w299]
          frame False {
          }
          frame True {
            n100 = Delete From Array(array=w299, length=600) -> (deleted portion=w297:dbl[])  [unwired: 1 in, 1 out]
            n101 = Array Max & Min(array=w297) -> (max value=w296:dbl, min value=w295:dbl)  [unwired: 2 out]
            n102 = Subtract(x=w296, y=w295) -> (x-y=w294:dbl)
            n103 = Less?(x=w294, y=2.0) -> (x < y?=w292:bool)
          }
        }
        "Temp stable" <- w279
        n104 = case shown="False" w279 {
          tunnel: w287 -> [w309 w320]
          tunnel: [w308 w320] -> w286
          tunnel: [w306 "" ("State(s) in Front (\"\")")] -> w285
          tunnel: w284 -> [w303 _]
          tunnel: w278 -> [w302 _]
          tunnel: w277 -> [w300 _]
          frame False {
            n105 = call "E-Time.vi"() -> ("Elapsed Time (sec)"=w310:dbl)  [unwired: 9 in, 2 out]
            n106 = call "Timeout Calc.vi"("Complete time"=w310, "Gather Data Period"=1000, "Start Time"=w303) -> ("Delay Time"=w305:i32)  [unwired: 8 in]
            n107 = event shown="[0] Timeout" {
              selector: _ -> [_]
              dyn-events: _ -> [_]
              timeout: w305 -> [_]
              tunnel: [w316] -> w307
              tunnel: [w315] -> w306
              tunnel: w302 -> [w313]
              tunnel: [w312] -> w301
              tunnel: w300 -> [w311]
              event Timeout {
                n108 = event-data() -> ()  [unwired: 1 in, 2 out]
                n109 = local read "Temperature-RDB"() -> (w314:dbl)
                n110 = case shown="True" w311 {
                  tunnel: ["Post Time\nGet Power\nCDAQ: Get Data\nWait for Temp Stable for 10 Min" ("State(s) in Front (\"\")") "Post Time\nGet Power\nAgilent: Get Data\nWait for Temp Stable for 10 Min" ("State(s) in Front (\"\")")] -> w315
                  frame True {
                  }
                  frame False {
                  }
                }
                n111 = call "E-Time.vi"() -> ("Elapsed Time (sec)"=w316:dbl)  [unwired: 9 in, 2 out]
                n112 = Build Array (concatenate)(w313, w314) -> (w312:dbl[])
              }
            }
            n113 = Bundle By Name(cluster=w309, "Tstart"=w307, "Temps"=w301) -> (w308:T6)
          }
          frame True {
          }
        }
        n114 = local write "String"("Air Fluffing...") -> ()
        n115 = call <vilib>:"Add State(s) to Queue__jki_lib_state_machine.vi"("State(s) in Front (\"\")"=w285, "State(s) in (\"\")"=w290) -> ("States Out"=w289:string)  [unwired: 13 in]
      }
      frame "Agilent: Save Set Channels" {
        w325 = "," ("string")
        w338 = "," ("string")
        # "Your code here.\n(You can make a copy of, or modify, this frame)"
        n116 = Unbundle By Name(w334) -> ("Equipment.Com Agilent"=w328:refnum<visa-resource-name>, "RDB Channel"=w332:string)
        n117 = global read "Global Test Variables DPT.vi" "Globals for Dryer Performance Test"() -> (w341:T8)
        n118 = global read "Global Test Variables DPT.vi" "34970 ChTemp Chan"() -> (w322:string)
        n119 = global read "Global Test Variables DPT.vi" "34970 RDB Chan"() -> (w324:string)
        n120 = global read "Global Test Variables DPT.vi" "34970 RH Chan"() -> (w323:string)
        n121 = Equal?(x=w328, y=refnum<visa-resource-name> "AGILENT-34980A" ("VISA resource name")) -> (x = y?=w326:bool)
        n122 = Unbundle By Name(w341) -> ("Agilent Setup.RH Chan"=w340:string, "Agilent Setup.Temp Chan"=w339:string)
        n123 = Concatenate Strings(w324, w325, w323, w325, w322) -> (w321:string)
        n124 = Concatenate Strings(w340, w338, w339, w338, w332) -> (w337:string)
        "Test AG Chan List" <- w337
        n125 = case shown="False" w326 {
          tunnel: w337 -> [_ w359]
          tunnel: [w348 w358] -> w335
          tunnel: w333 -> [w351 w357]
          tunnel: [w346 w354] -> w331
          tunnel: w328 -> [w352 w353]
          tunnel: w321 -> [w347 _]
          frame False {
            n126 = call "Read Scan List.vi"("error in (no error)"=w351, "VISA Resource Name"=w352) -> ("error out"=w349:errorcluster, "Scan List"=w348:string, "VISA Resource Name Out"=w344:refnum<visa-resource-name>)  [unwired: 7 in]
            n127 = call "Delay mS.vi"("Error In"=w349, "milliseconds to wait"=u32 500) -> ("Error Out"=w345:errorcluster)  [unwired: 13 in]
            n128 = call "Conf Scan List.vi"("Scan List (empty)"=w347, "error in (no error)"=w345, "VISA Resource Name"=w344) -> ("error out"=w346:errorcluster)  [unwired: 6 in, 2 out]
          }
          frame True {
            n129 = call "AG34980A Get Scan List.vi"("VISA resource name"=w353, "error in (no error)"=w357) -> ("Channel List"=w358:string, "error out"=w360:errorcluster)  [unwired: 11 in, 1 out]
            n130 = call "Delay mS.vi"("Error In"=w360, "milliseconds to wait"=u32 500) -> ("Error Out"=w356:errorcluster)  [unwired: 13 in]
            n131 = call "AG34980A Configure Scan.vi"("VISA resource name"=w353, "Scan List(empty)"=w359, "error in (no error)"=w356) -> ("error out"=w354:errorcluster)  [unwired: 11 in, 1 out]
          }
        }
        "Saved Channel List" <- w335
        n132 = Bundle By Name(cluster=w334, "Agilent Channel List"=w335) -> (w336:T6)
        n133 = call "Delay mS.vi"("Error In"=w331, "milliseconds to wait"=u32 1000) -> ("Error Out"=w330:errorcluster)  [unwired: 13 in]
        n134 = call <vilib>:"Add State(s) to Queue__jki_lib_state_machine.vi"("State(s) in (\"\")"=w343) -> ("States Out"=w342:string)  [unwired: 14 in]
      }
      frame "Init: Time" {
        # "Your code here.\n(You can make a copy of, or modify, this frame)"
        n135 = Unbundle By Name(w366) -> ("CDAQ Tasks"=w363:refnum<k21>[])  [unwired: 1 out]
        n136 = case shown="True" TRUE {
          tunnel: w365 -> [w373 w377]
          tunnel: [w373 w376] -> w364
          tunnel: w363 -> [w372 w375]
          tunnel: [w372 w374] -> w362
          frame False {
          }
          frame True {
            n137 = call "03 cDAQ Chan Tester.vi"("Tasks In"=w375, "error in (no error)"=w377, "Mode"=T3."Init CDAQ") -> ("error out"=w376:errorcluster, "Tasks Out"=w374:refnum<k21>[])  [unwired: 6 in, 1 out]
          }
        }
        n138 = call "E-Time.vi"("error in (no error)"=w364) -> ("error out"=w367:errorcluster, "Elapsed Time (sec)"=w368:dbl)  [unwired: 8 in, 1 out]
        n139 = Bundle By Name(cluster=w366, "CDAQ Tasks"=w362, "T0"=w368, "Tstart"=w368) -> (w369:T6)
        n140 = call <vilib>:"Add State(s) to Queue__jki_lib_state_machine.vi"("State(s) in (\"\")"=w371) -> ("States Out"=w370:string)  [unwired: 14 in]
      }
      frame "Agilent: Restore Channels" {
        # "Your code here.\n(You can make a copy of, or modify, this frame)"
        n141 = Unbundle By Name(w383) -> ("Equipment.Com Agilent"=w380:refnum<visa-resource-name>, "Agilent Channel List"=w382:string)
        n142 = Equal?(x=w380, y=refnum<visa-resource-name> "AGILENT-34980A" ("VISA resource name")) -> (x = y?=w379:bool)
        n143 = case shown="False" w379 {
          tunnel: w385 -> [w390 w395]
          tunnel: [w389 w394] -> w384
          tunnel: w382 -> [w391 w393]
          tunnel: w380 -> [w388 w392]
          frame False {
            n144 = call "Conf Scan List.vi"("Scan List (empty)"=w391, "error in (no error)"=w390, "VISA Resource Name"=w388) -> ("error out"=w389:errorcluster)  [unwired: 6 in, 2 out]
          }
          frame True {
            n145 = call "AG34980A Configure Scan.vi"("VISA resource name"=w392, "Scan List(empty)"=w393, "error in (no error)"=w395) -> ("error out"=w394:errorcluster)  [unwired: 11 in, 1 out]
          }
        }
        n146 = call <vilib>:"Add State(s) to Queue__jki_lib_state_machine.vi"("State(s) in (\"\")"=w387) -> ("States Out"=w386:string)  [unwired: 14 in]
      }
      frame "Agilent: Get Data" {
        # "Your code here.\n(You can make a copy of, or modify, this frame)"
        n147 = global read "Global Test Variables DPT.vi" "Globals for Dryer Performance Test"() -> (w399:T8)
        n148 = Unbundle By Name(w406) -> ("Equipment.Com Agilent"=w402:refnum<visa-resource-name>)
        n149 = Unbundle By Name(w399) -> ("Test Setup.RH-IP"=w396:string)
        "Test Setup.RH-IP" <- w396
        n150 = Equal?(x=w402, y=refnum<visa-resource-name> "AGILENT-34980A" ("VISA resource name")) -> (x = y?=w401:bool)
        n151 = Equal?(x=w396, y="0") -> (x = y?=w398:bool)
        n152 = case shown="False" w401 {
          tunnel: [w417 w447] -> w408
          tunnel: [w416 w446] -> w407
          tunnel: w405 -> [w419 w445]
          tunnel: [w415 w444] -> w404
          tunnel: w402 -> [w420 w443]
          tunnel: w398 -> [w414 _]
          tunnel: [w412 w442] -> w397
          tunnel: w396 -> [w411 _]
          frame False {
            n153 = call "Read Chans in Scan List.vi"("error in (no error)"=w419, "VISA Resource Name"=w420) -> ("error out"=w413:errorcluster, "Values Array"=w418:dbl[])  [unwired: 7 in, 1 out]
            n154 = case shown="False" w414 {
              tunnel: w418 -> [w425 w438]
              tunnel: [w422 w430] -> w417
              tunnel: [w421 w429] -> w416
              tunnel: [w424 w437] -> w415
              tunnel: w413 -> [w423 w436]
              tunnel: [w423 w435] -> w412
              tunnel: w411 -> [_ w434]
              frame True {
                n155 = Index Array(array=w425, index #1=1 ("index"), index #2=2 ("index"), index #3=0 ("index")) -> (element #1=w422:dbl, element #2=w421:dbl, element #3=w424:dbl)
              }
              frame False {
                n156 = call "Newport ITX-D3N.vi"("error in (no error)"=w436, "Machine"=w434) -> ("error out"=w435:errorcluster, "[Temp (F), RH]"=w433:dbl[])  [unwired: 8 in]
                n157 = Index Array(array=w438, index #1=1 ("index"), index #2=2 ("index"), index #3=0 ("index")) -> (element #3=w437:dbl)  [unwired: 2 out]
                n158 = Index Array(array=w433, index #1=1 ("index"), index #2=0 ("index")) -> (element #1=w430:dbl, element #2=w429:dbl)
              }
            }
          }
          frame True {
            n159 = call "AG34980A Initiate.vi"("VISA resource name"=w443, "error in (no error)"=w445) -> ("VISA resource name out"=w452:refnum<visa-resource-name>, "error out"=w450:errorcluster)  [unwired: 12 in]
            n160 = call "AG34980A Fetch.vi"("VISA resource name"=w452, "Numbers Only (T:On)"=TRUE, "error in (no error)"=w450) -> ("VISA resource name out"=w453:refnum<visa-resource-name>, "Output Data (Numbers Only)"=w449:dbl[], "error out"=w451:errorcluster)  [unwired: 8 in, 2 out]
            n161 = call "AG34980A Error Query (Multiple).vi"("VISA resource name"=w453, "error in (no error)"=w451) -> ("Error Message"=→"Agilent Error Message":string, "error out"=w442:errorcluster)  [unwired: 10 in, 2 out]
            n162 = Index Array(array=w449, index #1=0 ("index"), index #2=1 ("index"), index #3=2 ("index")) -> (element #1=w447:dbl, element #2=w446:dbl, element #3=w444:dbl)
          }
        }
        "RH" <- w408
        "Ambient Temp(F)" <- w407
        "RDB (F)" <- w404
        "Temperature-RDB" <- w404
        n163 = call <vilib>:"Add State(s) to Queue__jki_lib_state_machine.vi"("State(s) in (\"\")"=w410) -> ("States Out"=w409:string)  [unwired: 14 in]
      }
      frame "CDAQ: Get Data" {
        # "Your code here.\n(You can make a copy of, or modify, this frame)"
        n164 = global read "Global Test Variables DPT.vi" "Globals for Dryer Performance Test"() -> (w475:T8)
        n165 = Unbundle By Name(w466) -> ("CDAQ Tasks"=w465:refnum<k21>[])
        n166 = Unbundle By Name(w475) -> ("cDAQ Array Locations.RDB Channel"=w474:string, "cDAQ Array Locations.Temp Chan"=w469:string, "cDAQ Array Locations.RDB Channel"=w468:string, "cDAQ Array Locations.RH Chan"=w467:string, "Test Setup.RH-IP"=w461:string)
        n167 = local write "Test Setup.RH-IP"(w461) -> ()
        n168 = call "03 cDAQ Chan Tester.vi"("Tasks In"=w465, "error in (no error)"=w479, "Mode"=T3."Gather DATA") -> ("error out"=w464:errorcluster, "CDAQ Data Out"=w477:dbl[])  [unwired: 6 in, 1 out]
        "CDAQ Data Out" <- w477
        n169 = Decimal String To Number(string=w474) -> (number=w473:i32)  [unwired: 2 in, 1 out]
        n170 = Decimal String To Number(string=w469) -> (number=w472:i32)  [unwired: 2 in, 1 out]
        n171 = Decimal String To Number(string=w468) -> (number=w471:i32)  [unwired: 2 in, 1 out]
        n172 = Decimal String To Number(string=w467) -> (number=w470:i32)  [unwired: 2 in, 1 out]
        n173 = Index Array(array=w477, index #1=w473, index #2=w472, index #3=w471, index #4=w470) -> (element #1=w476:dbl, element #2=w462:dbl, element #3=w460:dbl, element #4=w459:dbl)
        n174 = case shown="\"any\", Default" w461 {
          tunnel: w461 -> [_ w486]
          tunnel: [w482 w485] -> w458
          tunnel: [w483 w484] -> w463
          tunnel: w462 -> [w483 _]
          tunnel: w459 -> [w482 _]
          frame "0" {
          }
          frame "any", Default {
            n175 = call "Newport ITX-D3N.vi"("Machine"=w486) -> ("[Temp (F), RH]"=w489:dbl[])  [unwired: 9 in, 1 out]
            n176 = Index Array(array=w489, index #1=0 ("index"), index #2=1 ("index")) -> (element #1=w484:dbl, element #2=w485:dbl)
          }
        }
        n177 = local write "RH"(w458) -> ()
        n178 = local write "Ambient Temp(F)"(w463) -> ()
        n179 = local write "RDB (F)"(w476) -> ()
        n180 = local write "Temperature-RDB"(w460) -> ()
        n181 = call <vilib>:"Add State(s) to Queue__jki_lib_state_machine.vi"("State(s) in (\"\")"=w481) -> ("States Out"=w480:string)  [unwired: 14 in]
      }
      frame "Get Cold Dryer Weight" {
        # "Your code here.\n(You can make a copy of, or modify, this frame)"
        n182 = for {
          N: 5 -> [_]
          tunnel: [w498] -> w491 mode=indexing
          shift-right: [w499] -> w493
          shift-left: w494 -> [w500]
          n183 = call "Weight Input.vi"("Error In"=w500) -> ("Ave in Median Range"=w498:dbl, "error out"=w499:errorcluster)  [unwired: 10 in, 3 out]
        }
        n184 = call-poly <vilib>:"Mean.vi"("X"=w491) -> ("mean"=→"Cold Dryer Weight":dbl)  [unwired: 1 out]
        n185 = call <vilib>:"Add State(s) to Queue__jki_lib_state_machine.vi"("State(s) in (\"\")"=w497) -> ("States Out"=w496:string)  [unwired: 14 in]
      }
      frame "Get Power" {
        # "Your code here.\n(You can make a copy of, or modify, this frame)"
        n186 = Unbundle By Name(w502) -> ("Equipment.Com Power Meter"=w506:refnum<visa-resource-name>)
        n187 = call "WT500 Read Power.vi"("VISA resource name"=w506, "WT500 CMDS"=WT500_Sequences."GetReadings", "error in (no error)"=w504) -> ("PowerData"=w505:T9, "error out"=w503:errorcluster)  [unwired: 7 in, 4 out]
        n188 = Unbundle By Name(w505) -> ("Power"=→"Power":dbl)
        n189 = call <vilib>:"Add State(s) to Queue__jki_lib_state_machine.vi"("State(s) in (\"\")"=w509) -> ("States Out"=w508:string)  [unwired: 14 in]
      }
      frame "Post Time" {
        # "Your code here.\n(You can make a copy of, or modify, this frame)"
        n190 = Unbundle By Name(w514) -> ("T0"=w512:dbl)
        n191 = call "E-Time.vi"() -> ("Elapsed Time (sec)"=w513:dbl)  [unwired: 9 in, 2 out]
        n192 = Subtract(x=w513, y=w512) -> (x-y=→"Timer":dbl)
        n193 = call <vilib>:"Add State(s) to Queue__jki_lib_state_machine.vi"("State(s) in (\"\")"=w516) -> ("States Out"=w515:string)  [unwired: 14 in]
      }
    }
    n194 = case shown="True" "Debug?" {
      tunnel: w14 -> [_ w32]
      tunnel: w12 -> [w29 w31]
      tunnel: [w29 w30] -> w13
      frame False {
      }
      frame True {
        n195 = Build Array (concatenate)(w31, w32) -> (w30:string[])
        "Debug State" <- w30
      }
    }
    n196 = local read "CDAQ?"() -> (w16:bool)
    n197 = case shown="True" "Exit" {
      tunnel: w19 -> [w33 w38]
      tunnel: [w33 w37] -> w18
      tunnel: w16 -> [_ w34]
      frame False {
      }
      frame True {
        n198 = case shown="False" w34 {
          tunnel: ["Get Cold Dryer Weight\nMacro: Exit" "Agilent: Restore Channels\nGet Cold Dryer Weight\nMacro: Exit"] -> w36
          frame True {
          }
          frame False {
          }
        }
        n199 = call <vilib>:"Add State(s) to Queue__jki_lib_state_machine.vi"("State(s) in Front (\"\")"=w36, "State(s) in (\"\")"=w38) -> ("States Out"=w37:string)  [unwired: 13 in]
        n200 = local write "Exit"(FALSE ("Exit")) -> ()
      }
    }
  }
  "Error Out" <- w2
